vi "Ramp SubVI FOR BENCHMARK.vi"   [LabVIEW 2011]
types:
  T1 = typedef "WPI_JoystickDevRef.ctl" = cluster{"Device":T2}
  T2 = typedef "WPI_JoystickDeviceEnum.ctl" = enum16{"USB 1", "USB 2", "USB 3", "USB 4", "Kinect 1", "Kinect 2"}
  T3 = cluster{"axis 1 (x)":dbl, "axis 2 (y)":dbl, "axis 3 (throttle)":dbl, "axis 4":dbl, "axis 5":dbl, "axis 6":dbl}
  T4 = typedef "WPI_DigitalInputDevRef.ctl" = cluster{"DevStatus":errorcluster, "DIO Channel":T5, "Digital Module":T6}
  T5 = typedef "FPGA_DIOChannel.ctl" = enum8{"DIO 1", "DIO 2", "DIO 3", "DIO 4", "DIO 5", "DIO 6", "DIO 7", "DIO 8", "DIO 9", "DIO 10", "DIO 11", "DIO 12", "DIO 13", "DIO 14", "Invalid"}
  T6 = typedef "FPGA_TypedefDigitalModule.ctl" = enum16{"Digital Module 1", "Digital Module 2"}
  T7 = typedef "WPI_MotorControlDeviceRef.ctl" = cluster{"DeviceStatus":errorcluster, "Type":enum16{"PWM", "CAN"}, "PWM":cluster{"Digital Module":T6, "PWM Channel":T8, "DeadBand":T9}, "CAN":cluster{"Device Number":u8, "Control Mode":T10, "Semaphore":T11, "Max Vout":dbl}, "Invert":bool, "TransformRef":T12, "InvTransformRef":T12}
  T8 = typedef "FPGA_DIOPWMChannel.ctl" = enum8{"PWM 1", "PWM 2", "PWM 3", "PWM 4", "PWM 5", "PWM 6", "PWM 7", "PWM 8", "PWM 9", "PWM 10", "Invalid"}
  T9 = typedef "WPI_PWMDeadband.ctl" = cluster{"Name":string, "maxPositivePwm":i32, "minPositivePwm":i32, "centerPwm":i32, "maxNegativePwm":i32, "minNegativePwm":i32, "angularRange":u16}
  T10 = typedef "WPI_CANJaguar_ControlMode.ctl" = enum8{"Percent VBus", "Current", "Speed", "Position", "Voltage"}
  T11 = typedef "Semaphore RefNum" = refnum<k1>
  T12 = typedef "WPI_PWMTransform_ConPane.ctl" = refnum<vi>
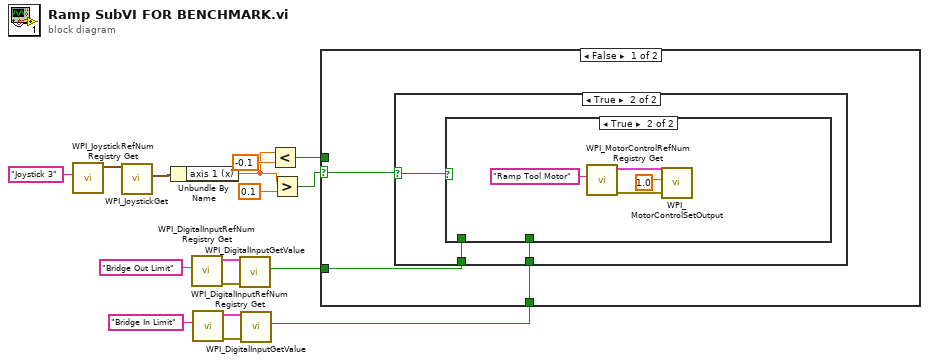
[diagram p0: block diagram]
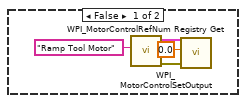
[diagram p2: hidden frame]
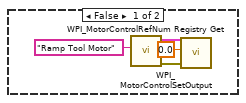
[diagram p3: hidden frame]
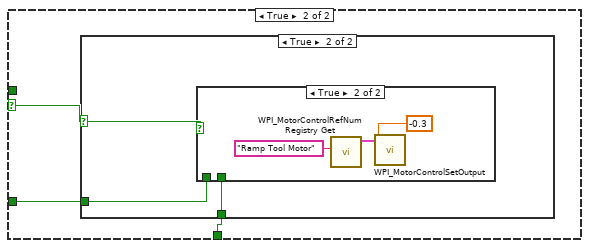
[diagram p4: hidden frame]
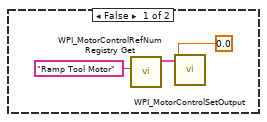
[diagram p5: hidden frame]
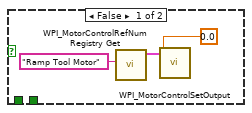
[diagram p6: hidden frame]
diagram:
  n1 = call <vilib>:"WPI_JoystickRefNum Registry Get.vi"("refnum name"="Joystick 3") -> ("JoystickDevRef"=w1:T1)  [unwired: 9 in, 1 out]
  n2 = call <vilib>:"WPI_JoystickGet.vi"("JoystickDevRef"=w1) -> ("Axes"=w3:T3)  [unwired: 4 in, 2 out]
  n3 = Unbundle By Name(w3) -> ("axis 1 (x)"=w4:dbl)
  n4 = call <vilib>:"WPI_DigitalInputRefNum Registry Get.vi"("refnum name"="Bridge Out Limit") -> ("error out"=w9:errorcluster, "DigitalInputDevRef"=w10:T4)  [unwired: 9 in]
  n5 = call <vilib>:"WPI_DigitalInputRefNum Registry Get.vi"("refnum name"="Bridge In Limit") -> ("error out"=w13:errorcluster, "DigitalInputDevRef"=w14:T4)  [unwired: 9 in]
  n6 = call <vilib>:"WPI_DigitalInputGetValue.vi"("error in (no error)"=w9, "DigitalInputDevRef"=w10) -> ("Value"=w11:bool)  [unwired: 7 in, 2 out]
  n7 = call <vilib>:"WPI_DigitalInputGetValue.vi"("error in (no error)"=w13, "DigitalInputDevRef"=w14) -> ("Value"=w16:bool)  [unwired: 7 in, 2 out]
  n8 = Less?(x=w4, y=-0.1) -> (x < y?=w7:bool)
  n9 = Greater?(x=w4, y=0.1) -> (0:w8:bool)
  n10 = case shown="False" w8 {
    selector: w8 -> [w17 w37]
    tunnel: w7 -> [_ _]
    tunnel: w11 -> [w19 w36]
    tunnel: w16 -> [w18 w35]
    frame False {
      n11 = case shown="True" w17 {
        selector: w17 -> [_ w24]
        tunnel: w19 -> [_ w26]
        tunnel: w18 -> [_ w25]
        frame False {
          n12 = call <vilib>:"WPI_MotorControlRefNum Registry Get.vi"("refnum name"="Ramp Tool Motor") -> ("error out"=w23:errorcluster, "MotorControlDevRef"=w22:T7)  [unwired: 9 in]
          n13 = call <vilib>:"WPI_MotorControlSetOutput.vi"("error in (no error)"=w23, "Output"=0.0, "MotorControlDevRef"=w22) -> ()  [unwired: 7 in, 2 out]
        }
        frame True {
          n14 = case shown="True" w24 {
            tunnel: w26 -> [_ _]
            tunnel: w25 -> [_ _]
            frame False {
              n15 = call <vilib>:"WPI_MotorControlRefNum Registry Get.vi"("refnum name"="Ramp Tool Motor") -> ("error out"=w30:errorcluster, "MotorControlDevRef"=w29:T7)  [unwired: 9 in]
              n16 = call <vilib>:"WPI_MotorControlSetOutput.vi"("error in (no error)"=w30, "Output"=0.0, "MotorControlDevRef"=w29) -> ()  [unwired: 7 in, 2 out]
            }
            frame True {
              n17 = call <vilib>:"WPI_MotorControlRefNum Registry Get.vi"("refnum name"="Ramp Tool Motor") -> ("error out"=w34:errorcluster, "MotorControlDevRef"=w33:T7)  [unwired: 9 in]
              n18 = call <vilib>:"WPI_MotorControlSetOutput.vi"("error in (no error)"=w34, "Output"=1.0, "MotorControlDevRef"=w33) -> ()  [unwired: 7 in, 2 out]
            }
          }
        }
      }
    }
    frame True {
      n19 = case shown="True" w37 {
        selector: w37 -> [_ w43]
        tunnel: w36 -> [_ w42]
        tunnel: w35 -> [_ w41]
        frame False {
          n20 = call <vilib>:"WPI_MotorControlRefNum Registry Get.vi"("refnum name"="Ramp Tool Motor") -> ("MotorControlDevRef"=w40:T7)  [unwired: 9 in, 1 out]
          n21 = call <vilib>:"WPI_MotorControlSetOutput.vi"("Output"=0.0, "MotorControlDevRef"=w40) -> ()  [unwired: 8 in, 2 out]
        }
        frame True {
          n22 = case shown="True" w43 {
            tunnel: w42 -> [_ _]
            tunnel: w41 -> [_ _]
            frame False {
              n23 = call <vilib>:"WPI_MotorControlRefNum Registry Get.vi"("refnum name"="Ramp Tool Motor") -> ("MotorControlDevRef"=w46:T7)  [unwired: 9 in, 1 out]
              n24 = call <vilib>:"WPI_MotorControlSetOutput.vi"("Output"=0.0, "MotorControlDevRef"=w46) -> ()  [unwired: 8 in, 2 out]
            }
            frame True {
              n25 = call <vilib>:"WPI_MotorControlRefNum Registry Get.vi"("refnum name"="Ramp Tool Motor") -> ("MotorControlDevRef"=w49:T7)  [unwired: 9 in, 1 out]
              n26 = call <vilib>:"WPI_MotorControlSetOutput.vi"("Output"=-0.3, "MotorControlDevRef"=w49) -> ()  [unwired: 8 in, 2 out]
            }
          }
        }
      }
    }
  }
